vi "PC2_PROYECTO.vi"() -> ()   [LabVIEW 2016]
panel:
  in  "VariableSTR2":string
  in  "VariableDBL2":dbl
  in  "VariableBOOL2":bool
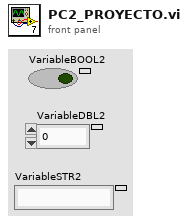
[diagram p1: front panel]
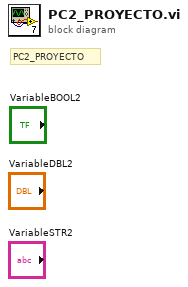
[diagram p0: block diagram]
diagram:
  # "PC2_PROYECTO"
